vi "GV_TakePhoto.vi"() -> ()   [LabVIEW 2023]
panel:
  out "Boolean":bool
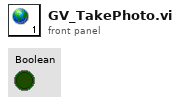
[diagram p1: front panel]
diagram:
